vi "Global - Configuration Options.vi"() -> ()   [LabVIEW 2017]
uses:
  <vilib>/h/FPGA/cRIO/shared/nicrio_ModuleControls/nicrio_cRIO-9234_DataRatesRing2.ctl
panel:
  in  "Chatter Data":T1={"Tool data"={"Number of teeth"=0.0}, "Cutting data"={"rpm"=0.0}, "Limits"={"Magnitude threshold"=0.0, "Tolerance"=2.0}, "G1 status"={"G1 trigger"=FALSE}}
  in  "Max Acceleration Threshold (g)":sgl=50.0
  in  "# of Channels":u32=11
  in  "Data Rate (Hz)":dbl=10240.0
  in  "Data Rate (kS/s)":T2=5 items=["51.200 kS/s (NI 9234)"=1, "25.600 kS/s (NI 9234)"=2, "17.067 kS/s (NI 9234)"=3, "12.800 kS/s (NI 9234)"=4, "10.240 kS/s (NI 9234)"=5, "8.533 kS/s (NI 9234)"=6, "7.314 kS/s (NI 9234)"=7, "6.400 kS/s (NI 9234)"=8, "5.689 kS/s (NI 9234)"=9, "5.120 kS/s (NI 9234)"=10, "4.654 kS/s (NI 9234)"=11, "4.267 kS/s (NI 9234)"=12, "3.938 kS/s (NI 9234)"=13, "3.657 kS/s (NI 9234)"=14, "3.413 kS/s (NI 9234)"=15, "3.200 kS/s (NI 9234)"=16, "3.012 kS/s (NI 9234)"=17, "2.845 kS/s (NI 9234)"=18, "2.695 kS/s (NI 9234)"=19, "2.560 kS/s (NI 9234)"=20, "2.438 kS/s (NI 9234)"=21, "2.328 kS/s (NI 9234)"=22, "2.226 kS/s (NI 9234)"=23, "2.133 kS/s (NI 9234)"=24, "2.048 kS/s (NI 9234)"=25, "1.969 kS/s (NI 9234)"=26, "1.896 kS/s (NI 9234)"=27, "1.829 kS/s (NI 9234)"=28, "1.765 kS/s (NI 9234)"=29, "1.707 kS/s (NI 9234)"=30, "1.652 kS/s (NI 9234)"=31]
  in  "Acceleration Log Folder":path=path "/home/lvuser/Log/logfiles_deploy"
  in  "Error Log Duplicate Interval (ms)":u32=5000
  in  "Network Stream Polling Timeout (ms)":i32=500
  in  "Debugging":bool=TRUE
  in  "Error Log Max Size (bytes)":i64=100000
  in  "RT Error Log":path=path "/home/lvuser/Log/error_log.txt"
  in  "PID Loop Period (us)":u32=200
  in  "Timeout Period (ticks)":u64=40000000
  in  "RT Stream Name":string="FanControlSampleProject_Command Stream from RT"
  in  "Monitoring Loop Rate (ms)":u32=500
  in  "Watchdog Pet Rate (ms)":u32=100
  in  "UI Stream Name":string="FanControlSampleProject_Command Stream from UI"
  in  "Network Stream Connect Timeout (ms)":i32=5000
  # "If you change any of these default configuration options, you must select Edit > Make Current Values Default before saving this VI."
  # "Make sure both of these match.\nData Rate (Hz) = Data Rate (kS/s) * 1000"
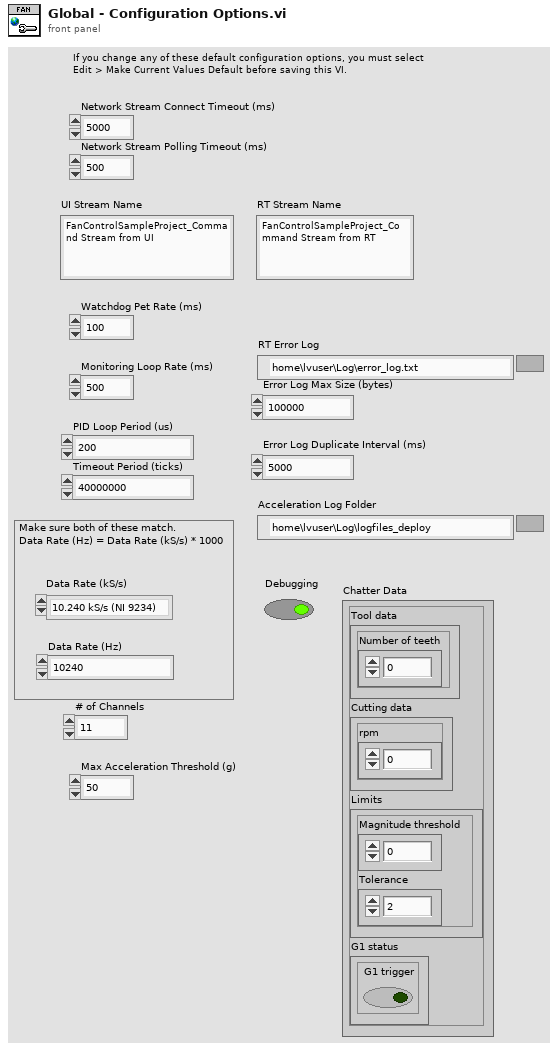
[diagram p1: front panel]
types:
  T1 = cluster{"Tool data":cluster{"Number of teeth":sgl}, "Cutting data":cluster{"rpm":sgl}, "Limits":cluster{"Magnitude threshold":sgl, "Tolerance":sgl}, "G1 status":cluster{"G1 trigger":bool}}
  T2 = typedef "nicrio_cRIO-9234_DataRatesRing2.ctl" = u8
diagram:
